vi "FlatToRichnixnet_grpc_ReadSignalXYRequest.vi"(5 "OutputClusterType":T1, 11 "InputCluster":T3) -> (3 "OutputCluster":T1)   [LabVIEW 2025, in "grpc-xnet_client.lvlib"]
uses:
  nixnet_grpc_ReadSignalXYRequest_Flat.ctl
  nidevice_grpc_Session_Flat.ctl
  nixnet_grpc_ReadSignalXYRequest.ctl
  nidevice_grpc_Session.ctl
  grpc-xnet_client.lvlib
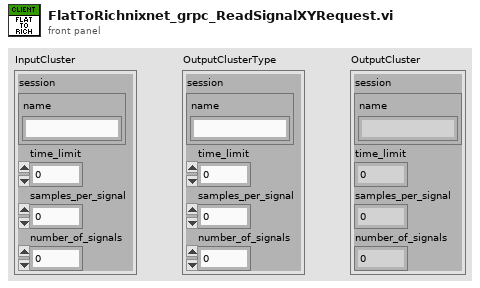
[diagram p1: front panel]
types:
  T1 = typedef "grpc-xnet_client.lvlib/nixnet_grpc_ReadSignalXYRequest.ctl" = cluster{"session":T2, "time_limit":u64, "samples_per_signal":u32, "number_of_signals":u32}
  T2 = typedef "grpc-xnet_client.lvlib/nidevice_grpc_Session.ctl" = cluster{"name":string}
  T3 = typedef "grpc-xnet_client.lvlib/nixnet_grpc_ReadSignalXYRequest_Flat.ctl" = cluster{"session":T4, "time_limit":u64, "samples_per_signal":u32, "number_of_signals":u32}
  T4 = typedef "grpc-xnet_client.lvlib/nidevice_grpc_Session_Flat.ctl" = cluster{"name":string}
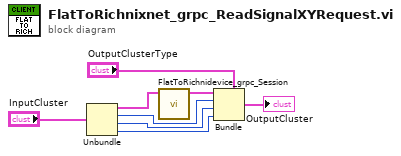
[diagram p0: block diagram]
diagram:
  n1 = Unbundle "Unbundle"("InputCluster") -> ("session"=w5:T4, "time_limit"=w3:u64, "samples_per_signal"=w2:u32, "number_of_signals"=w1:u32)
  n2 = call "FlatToRichnidevice_grpc_Session.vi"("InputCluster"=w5) -> ("OutputCluster"=w4:T2)  [unwired: 10 in]
  n3 = Bundle "Bundle"(cluster="OutputClusterType", "session"=w4, "time_limit"=w3, "samples_per_signal"=w2, "number_of_signals"=w1) -> (→"OutputCluster":T1)
